vi "Read from OPC Server2.vi"() -> ()   [LabVIEW 2017]
panel:
  in  "Stop Button":bool
  out "Numeric Control":dbl=22.0
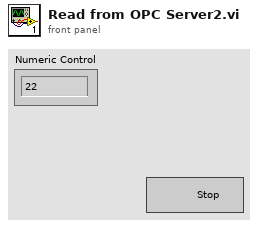
[diagram p1: front panel]
types:
  T1 = enum16{"Read", "Write", "ReadWrite", "BufferedRead", "BufferedReadWrite"}
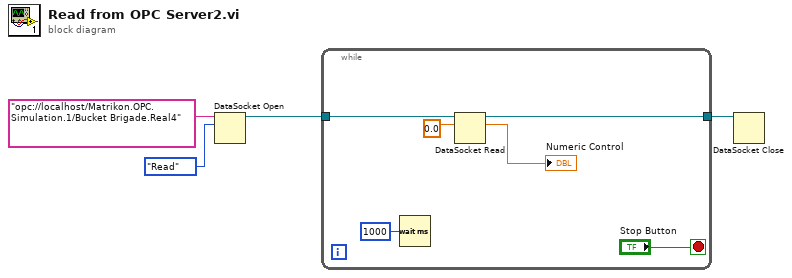
[diagram p0: block diagram]
diagram:
  n1 = DataSocket Open(10:T1."Read" ("mode"), 11:"opc://localhost/Matrikon.OPC.Simulation.1/Bucket Brigade.Real4" ("OPC URL")) -> (3:w4:refnum<k13>)  [unwired: 2 in, 1 out]
  n2 = while {
    tunnel: w4 -> [w8]
    tunnel: [w7] -> w3
    stop <- "Stop Button" stop-if-true
    n3 = Wait (ms)(milliseconds to wait=u32 1000) -> ()  [unwired: 1 out]
    n4 = DataSocket Read(10:0.0 ("Numeric Control"), 11:w8) -> (2:→"Numeric Control":dbl, 3:w7:refnum<k13>)  [unwired: 3 in, 5 out]
  }
  n5 = DataSocket Close(11:w3) -> ()  [unwired: 2 in, 2 out]
